vi "clearpath_parse_differential_speed.vi"(5 "ClearpathComm":T1) -> (0 "Left Speed":dbl, 1 "Right Speed":dbl, 2 "Left Accel":dbl, 3 "Right Accel":dbl, 4 "Data Valid?":bool=TRUE)   [LabVIEW 2012, in "clearpath_interface.lvlib"]
doc: "Parses differential speed data (Message type 0x8200)"
uses:
  clearpath_interface.lvlib
  cwrap_crio.dll
panel:
  # "Differential Speeds"
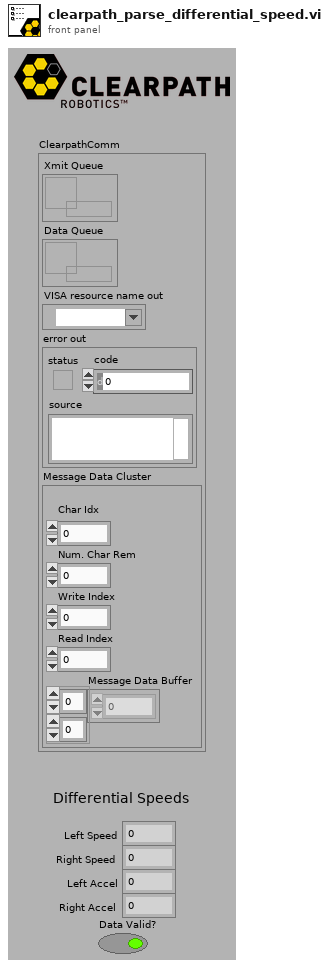
[diagram p1: front panel]
types:
  T1 = cluster{"Xmit Queue":refnum<queue>, "Data Queue":refnum<queue>, "VISA resource name out":refnum<visa-resource-name>, "error out":errorcluster, "Message Data Cluster":cluster{"\nChar Idx":u8, "Num. Char Rem":u8, "Write Index":u8, "Read Index":u8, "Message Data Buffer":u8[][]}}
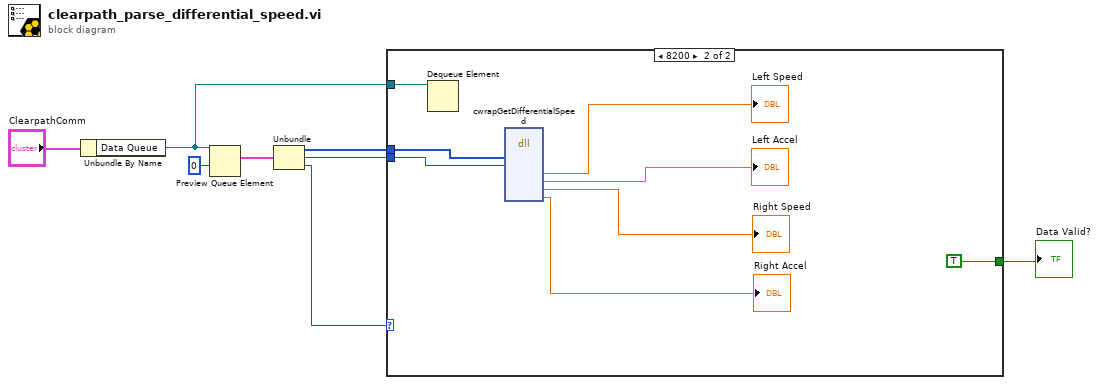
[diagram p0: block diagram]
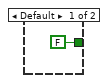
[diagram p2: hidden frame]
diagram:
  n1 = Unbundle By Name("ClearpathComm") -> ("Data Queue"=w1:refnum<queue>)
  n2 = Preview Queue Element(queue=w1, timeout in ms (-1)=0) -> (element=w6:cluster{u8[], "Length":i32, "Type":i32})  [unwired: 1 in, 3 out]
  n3 = Unbundle(w6) -> (w3:u8[], "Length"=w4:i32, "Type"=w5:i32)
  n4 = case shown="8200" w5 {
    tunnel: w4 -> [_ w12]
    tunnel: w3 -> [_ w13]
    tunnel: [FALSE TRUE] -> w2
    tunnel: w1 -> [_ w10]
    frame Default {
    }
    frame 33280 {
      n5 = Dequeue Element(queue=w10) -> ()  [unwired: 2 in, 4 out]
      n6 = dll-call lib="C:/Users/tebbeam/Documents/GitHub/IGVC-2013/Code/Project 1.0/Motors/Husky/cwrap_cRIO.*" fn="cwrapGetDifferentialSpeed"("packet"=w13, "len"=w12) -> ("l_speed"=→"Left Speed":dbl, "l_accel"=→"Left Accel":dbl, "r_speed"=→"Right Speed":dbl, "r_accel"=→"Right Accel":dbl)  [unwired: 10 in, 2 out]
    }
  }
  "Data Valid?" <- w2
